vi "Set Variant Property.vi"(6 "Control Ref Queue":T1, 8 "error in (no error)":errorcluster, 10 "Property In":variant, 11 "3D Bar.lvclass in":refnum<class "3D Bar.lvclass">) -> (0 "error out":errorcluster, 3 "3D Bar.lvclass":refnum<class "3D Bar.lvclass">)   [LabVIEW 2020, in "3D Bar.lvclass"]
uses:
  <vilib>/Math Plots/3D Math Plots/3D Bar/3D Bar/3D Bar.lvclass
  <vilib>/Math Plots/3D Math Plots/3D Bar/3D Bar/Typedef/3D Bar Property Array.ctl
  <vilib>/Math Plots/3D Math Plots/3D Bar/3D Bar/Typedef/3D Bar Property.ctl
  <vilib>/Math Plots/3D Math Plots/3D Plot/3D Plot/Typedef/Line Type.ctl
  <vilib>/Math Plots/3D Math Plots/3D Plot/Action String/3DMathPlot Ctrl Act Queue.ctl
  <vilib>/Math Plots/3D Math Plots/3D Plot/Action String/3DMathPlot Ctrl Act Cluster.ctl
  <vilib>/Math Plots/3D Math Plots/3D Plot/Action String/3DMathPlot State Class.ctl
  <vilib>/Math Plots/3D Math Plots/3D Bar/3D Bar/3D Bar.lvclass/3D Bar.ctl
  <vilib>/Math Plots/3D Math Plots/3D Plot/3D Plot/3D Plot.lvclass
panel:
  in  "3D Bar Property Array":T2
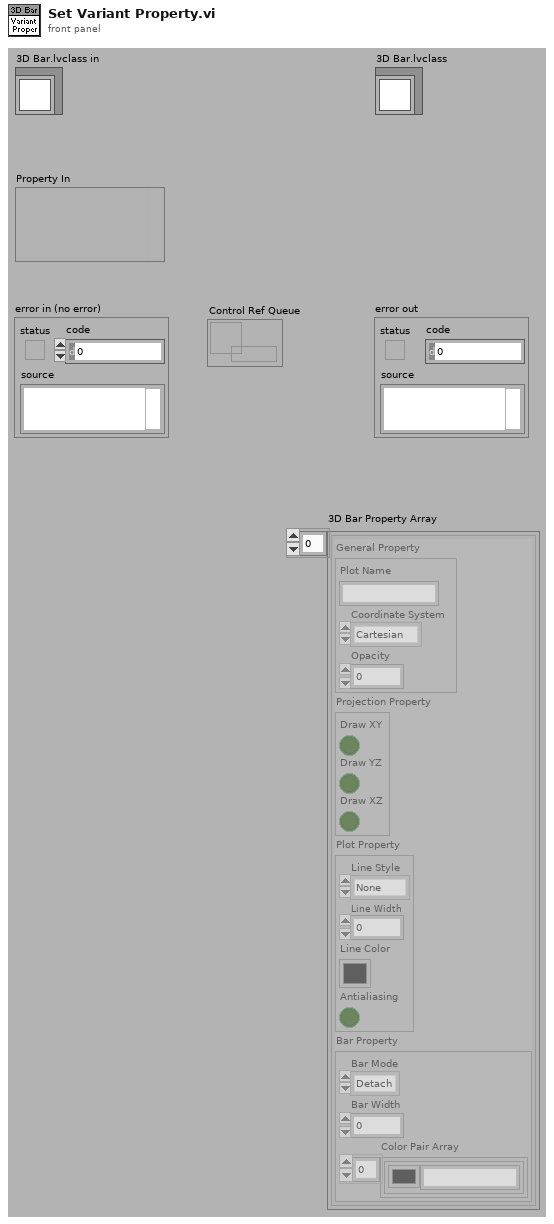
[diagram p1: front panel]
types:
  T1 = typedef "3DMathPlot Ctrl Act Queue.ctl" = refnum<queue>
  T2 = typedef "3D Bar.lvclass/3D Bar Property Array.ctl" = T3[]
  T3 = typedef "3D Bar.lvclass/3D Bar Property.ctl" = cluster{"General Property":cluster{"Plot Name":string, "Coordinate System":enum16{"Cartesian", "Cylindrical", "Spherical"}, "Opacity":sgl}, "Projection Property":cluster{"Draw XY":bool, "Draw YZ":bool, "Draw XZ":bool}, "Plot Property":cluster{"Line Style":T4, "Line Width":sgl, "Line Color":u32, "Antialiasing":bool}, "Bar Property":cluster{"Bar Mode":enum16{"Detach", "Group", "Stack"}, "Bar Width":sgl, "Color Pair Array":cluster{"Color":u32, "String":string}[]}}
  T4 = typedef "3D Plot.lvclass/Line Type.ctl" = enum16{"None", "Solid", "Dash", "Dot", "Dash Dot"}
  T5 = typedef "3DMathPlot State Class.ctl" = enum16{"Update All Objects (Undo)", "Update Light Object Only", "Update Axis Object Only", "Update Plot Object Only", "Update Cursor Object Only", "Update Axis Plot Cursor Objects", "No Update"}
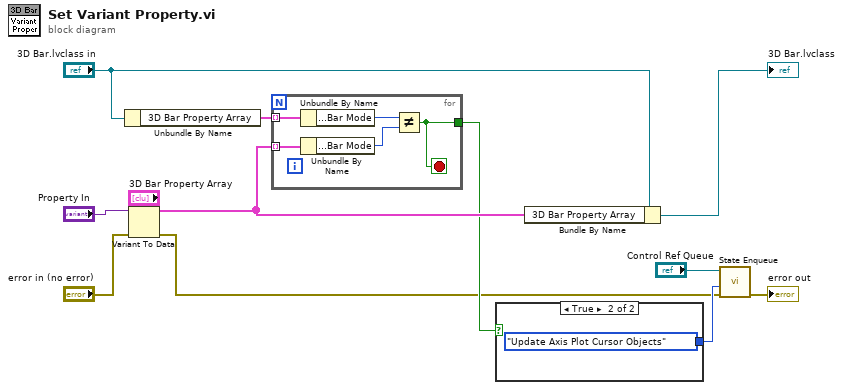
[diagram p0: block diagram]
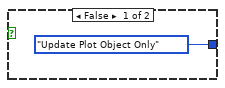
[diagram p2: hidden frame]
diagram:
  n1 = Unbundle By Name("3D Bar.lvclass in") -> ("3D Bar Property Array"=w5:T2)
  n2 = Variant To Data(error in="error in (no error)", type="3D Bar Property Array", Variant="Property In") -> (data=w6:T2, error out=w2:errorcluster)
  n3 = for {
    tunnel: w6 -> [w16] mode=indexing
    tunnel: w5 -> [w17] mode=indexing
    tunnel: [w13] -> w4
    stop <- w13 stop-if-true
    n4 = Unbundle By Name(w17) -> ("Bar Property.Bar Mode"=w15:enum16{"Detach", "Group", "Stack"})
    n5 = Unbundle By Name(w16) -> ("Bar Property.Bar Mode"=w14:enum16{"Detach", "Group", "Stack"})
    n6 = Not Equal?(x=w15, y=w14) -> (x != y?=w13:bool)
  }
  n7 = case shown="True" w4 {
    tunnel: [3DMathPlot_State_Class."Update Plot Object Only" ("Display State Change Class") 3DMathPlot_State_Class."Update Axis Plot Cursor Objects" ("Display State Change Class")] -> w3
    frame False {
    }
    frame True {
    }
  }
  n8 = Bundle By Name(cluster="3D Bar.lvclass in", "3D Bar Property Array"=w6) -> (→"3D Bar.lvclass":refnum<class "3D Bar.lvclass">)
  n9 = call <vilib>:"State Enqueue.vi"("error in (no error)"=w2, "Display State Change Class"=w3, "Control Ref Queue"="Control Ref Queue") -> ("error out"=→"error out":errorcluster)  [unwired: 8 out]
